vi "CreateWO-GetPartNumbers.vi"(5 "Parts Numbers and Descriptions":string[][](array[string]), 7 "Parts Numbers":string[](array[string]), 8 "error in (no error)":errorcluster, 11 "ERP-CreateWorkOrder in":refnum<class "ERP-CreateWorkOrder.lvclass">) -> (0 "error out":errorcluster, 3 "ERP-CreateWorkOrder out":refnum<class "ERP-CreateWorkOrder.lvclass">)   [LabVIEW 2013, in "ERP-CreateWorkOrder.lvclass"]
uses:
  ERP-CreateWorkOrder.lvclass
  ERP-CreateWorkOrder.lvclass/ERP-CreateWorkOrder.ctl
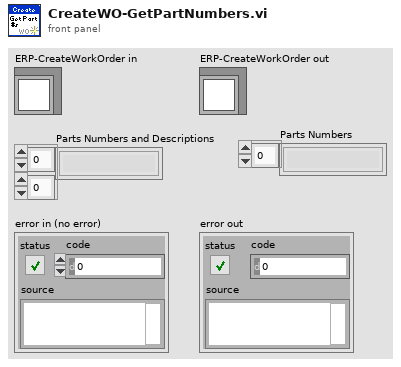
[diagram p1: front panel]
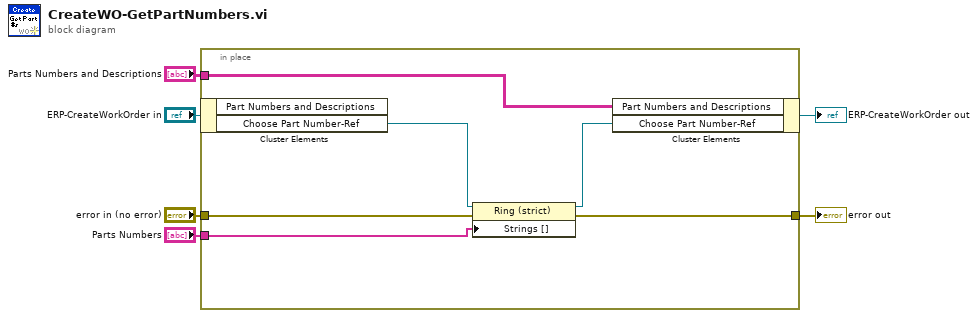
[diagram p0: block diagram]
diagram:
  n1 = in-place {
    in-place-border: "error in (no error)" -> [w11]
    in-place-border: [w10] -> w4
    in-place-border: "Parts Numbers and Descriptions" -> [w8]
    in-place-border: "Parts Numbers" -> [w7]
    n2 = in-place-cluster #1("ERP-CreateWorkOrder in") -> ("Choose Part Number-Ref"=w12:refnum<vi>)  [unwired: 1 out]
    n3 = property class="Ring (strict)"(reference=w12, error in=w11, "Strings []"=w7) -> (reference out=w9:refnum<vi>, error out=w10:errorcluster)
    n4 = in-place-cluster #1("Part Numbers and Descriptions"=w8, "Choose Part Number-Ref"=w9) -> (→"ERP-CreateWorkOrder out":refnum<class "ERP-CreateWorkOrder.lvclass">)
  }
  "error out" <- w4
